vi "AlliGator SS2 mat #Datasets Dialog with Skip Option.vi"(6 "Do not show this dialog again":bool, 10 "# Repetitions":i32) -> (0 "All?":bool, 1 "Cancel?":bool, 2 "Dataset to Show (-1: all)":i32, 4 "Do not show this dialog again?":bool)   [LabVIEW 2021, in "AlliGator Files.lvlib"]
uses:
  AlliGator Files.lvlib
  <vilib>/Utility/miscctls.llb/LVMinMaxIncTypeDef.ctl
panel:
  in  "Cancel":bool
  in  "Dataset to Show (-1: all)":i32=-1
  in  "Single":bool
  in  "All":bool
  out "Displayed Message":string
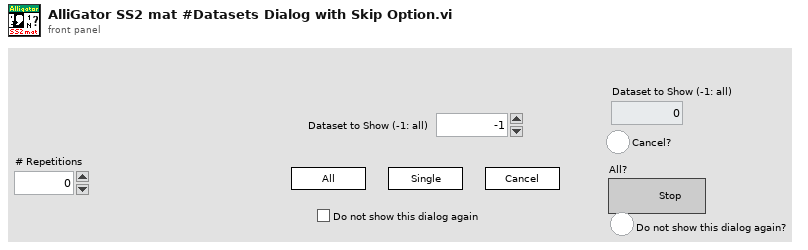
[diagram p1: front panel]
types:
  T1 = typedef "LVMinMaxIncTypeDef.ctl" = cluster{"Minimum":dbl, "Maximum":dbl, "Increment":dbl}
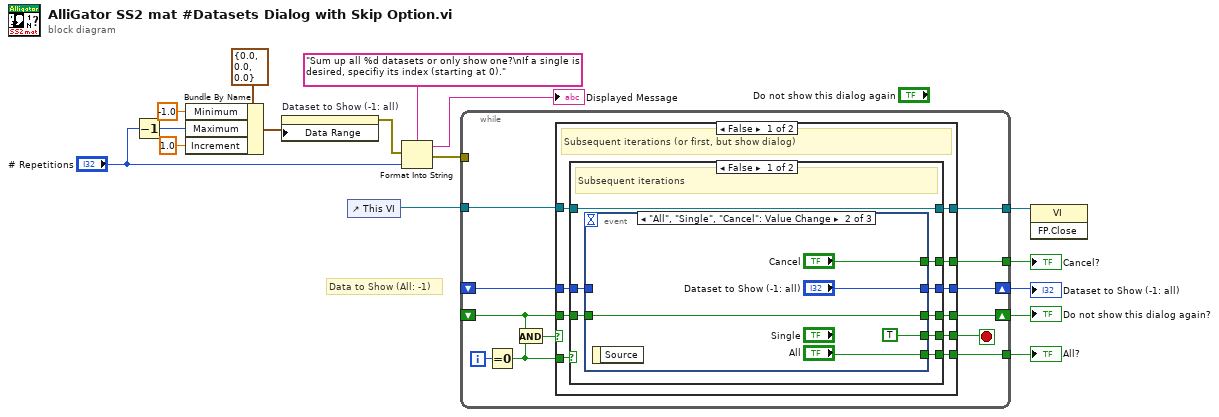
[diagram p0: block diagram]
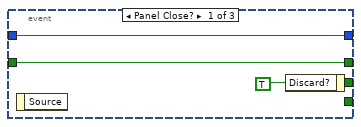
[diagram p2: hidden frame]
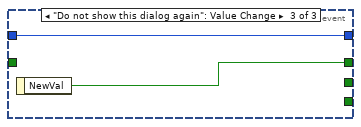
[diagram p3: hidden frame]
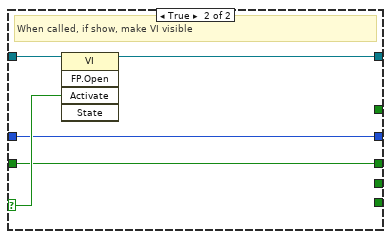
[diagram p4: hidden frame]
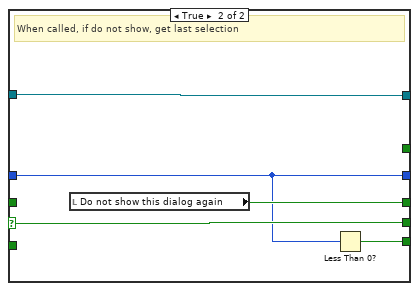
[diagram p5: hidden frame]
diagram:
  # "Data to Show (All: -1)"
  n1 = Decrement(x="# Repetitions") -> (x-1=w9:i32)
  n2 = Bundle By Name(cluster=T1 {"Minimum"=0.0, "Maximum"=0.0, "Increment"=0.0} ("Data Entry Limits"), "Minimum"=-1.0, "Maximum"=w9, "Increment"=1.0) -> (w11:T1)
  n3 = property on="Dataset to Show (-1: all)" class="DigNum (strict)"("Data Range"=w11) -> (error out=w7:errorcluster)  [unwired: 2 in, 1 out]
  n4 = control-ref of="This VI"() -> (w1:refnum<vi>)
  n5 = Format Into String(format string="Sum up all %d datasets or only show one?\nIf a single is desired, specifiy its index (starting at 0).", error in=w7, "# Repetitions") -> (resulting string=→"Displayed Message":string, error out=w6:errorcluster)  [unwired: 1 in]
  n6 = while {
    shift-right: [w28] -> w2
    shift-left: _ -> [w26]
    tunnel: w1 -> [w22]
    tunnel: [w21] -> w16
    tunnel: [w20] -> w15
    tunnel: w6 -> [_]
    shift-right: [w19] -> w4
    shift-left: _ -> [w18]
    tunnel: [w17] -> w3
    i -> [w27]
    stop <- w24 stop-if-true
    n7 = Equal To 0?(x=w27) -> (x = 0?=w23:bool)
    n8 = And(x=w26, y=w23) -> (x .and. y?=w25:bool)
    n9 = case shown="False" w25 {
      selector: w25 -> [_ w66]
      tunnel: [w38 w66] -> w24
      tunnel: [w37 w64] -> w28
      tunnel: w26 -> [w36 _]
      tunnel: w23 -> [w35 _]
      tunnel: w22 -> [w34 w65]
      tunnel: [w33 w65] -> w21
      tunnel: [w32 w62] -> w20
      tunnel: [w31 w63] -> w19
      tunnel: w18 -> [w30 w63]
      tunnel: [w29 _] -> w17
      frame False {
        # "Subsequent iterations (or first, but show dialog)"
        n10 = case shown="False" w35 {
          selector: w35 -> [_ w60]
          tunnel: [w46 _] -> w38
          tunnel: [w45 w58] -> w37
          tunnel: w36 -> [w44 w58]
          tunnel: w34 -> [w43 w61]
          tunnel: [w43 w59] -> w33
          tunnel: [w42 _] -> w32
          tunnel: [w41 w57] -> w31
          tunnel: w30 -> [w40 w57]
          tunnel: [w39 _] -> w29
          frame False {
            # "Subsequent iterations"
            n11 = event shown="[1] \"All\", \"Single\", \"Cancel\": Value Change" {
              selector: _ -> [_ _ _]
              dyn-events: _ -> [_ _ _]
              timeout: _ -> [_ _ _]
              tunnel: [w49 TRUE ("Discard?") _] -> w46
              tunnel: [w47 w50 w56] -> w45
              tunnel: w44 -> [w47 w50 _]
              tunnel: [_ "All" _] -> w42
              tunnel: [w48 "Dataset to Show (-1: all)" w55] -> w41
              tunnel: w40 -> [w48 _ w55]
              tunnel: [_ "Cancel" _] -> w39
              event Panel Close? {
                w49 = TRUE ("Discard?")
                n12 = event-data() -> ()  [unwired: 1 in, 1 out]
                n13 = event-data("Discard?"=w49) -> ()  [unwired: 1 in, 1 out]
              }
              event "All", "Single", "Cancel": Value Change {
                n14 = event-data() -> ()  [unwired: 1 in, 1 out]
              }
              event "Do not show this dialog again": Value Change {
                n15 = event-data() -> ("NewVal"=w56:bool)  [unwired: 1 in]
              }
            }
          }
          frame True {
            # "When called, if show, make VI visible"
            n16 = invoke class="VI" method="FP.Open"(reference=w61, "Activate"=w60) -> (reference out=w59:refnum<vi>)  [unwired: 3 in, 4 out]
          }
        }
      }
      frame True {
        # "When called, if do not show, get last selection"
        n17 = local read "Do not show this dialog again"() -> (w64:bool)
        n18 = Less Than 0?(x=w63) -> (x < 0?=w62:bool)
      }
    }
  }
  "All?" <- w15
  "Dataset to Show (-1: all)" <- w4
  "Cancel?" <- w3
  "Do not show this dialog again?" <- w2
  n19 = invoke class="VI" method="FP.Close"(reference=w16) -> ()  [unwired: 2 in, 3 out]
